vi "test_CSV.vi"() -> ()   [LabVIEW 2017]
uses:
  UI Error Handlers/support/Logging/Logging.lvlib
panel:
  out "appended path":path
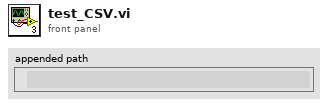
[diagram p1: front panel]
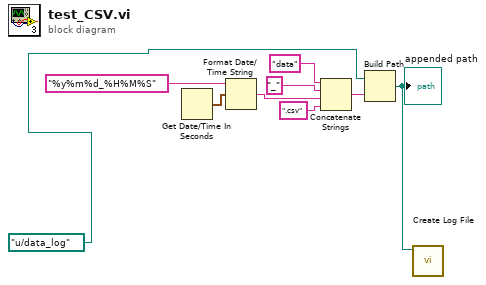
[diagram p0: block diagram]
diagram:
  n1 = Get Date/Time In Seconds() -> (seconds since 1Jan1904=w5:timestamp)
  n2 = Format Date/Time String(time format string (%c)="%y%m%d_%H%M%S", seconds (now)=w5) -> (date/time string=w8:string)  [unwired: 1 out]
  n3 = Concatenate Strings("data" ("string"), "_" ("string"), w8, ".csv" ("string")) -> (w3:string)
  n4 = Build Path(base path=path "u:/data_log" ("AVI Path"), name or relative path=w3) -> (appended path=w1:path)
  "appended path" <- w1
  n5 = call "Create Log File.vi"("Acceleration Exceeded Log Folder"=w1) -> ()  [unwired: 9 in, 2 out]
